vi "ConnectToISU.vi"(0 "ClientRef_In":refnum<k24>, 5 "error in (no error)":errorcluster, 6 "hostName":string="localhost", 8 "portNum":i32=50501, 9 "Get FWver(t)":bool, 11 "RunStartTest(T)":bool) -> (10 "StartTest?(P/F)":bool, 12 "GetVersion":string, 14 "ClientRef_out":refnum<k24>, 16 "ElapsedTime(s)":dbl format="%#.6g", 19 "error out":errorcluster)   [LabVIEW 2018]
uses:
  C:/RageATE-Tetra/Support/TetraLabGUI/FieldTestClient.dll
  Support/TetraLabGUI/FieldTestClient.dll
panel:
  out "FwVer(str)":string
  out "NaN/Path/Refnum?":bool
  out "StartTime":dbl format="%#.6f"
  out "Close?":bool
  out "isu_connected?(t)":bool
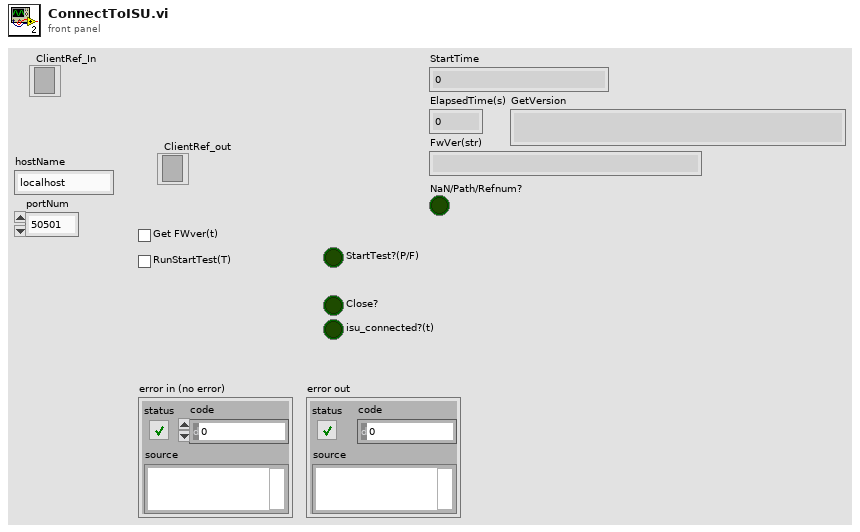
[diagram p1: front panel]
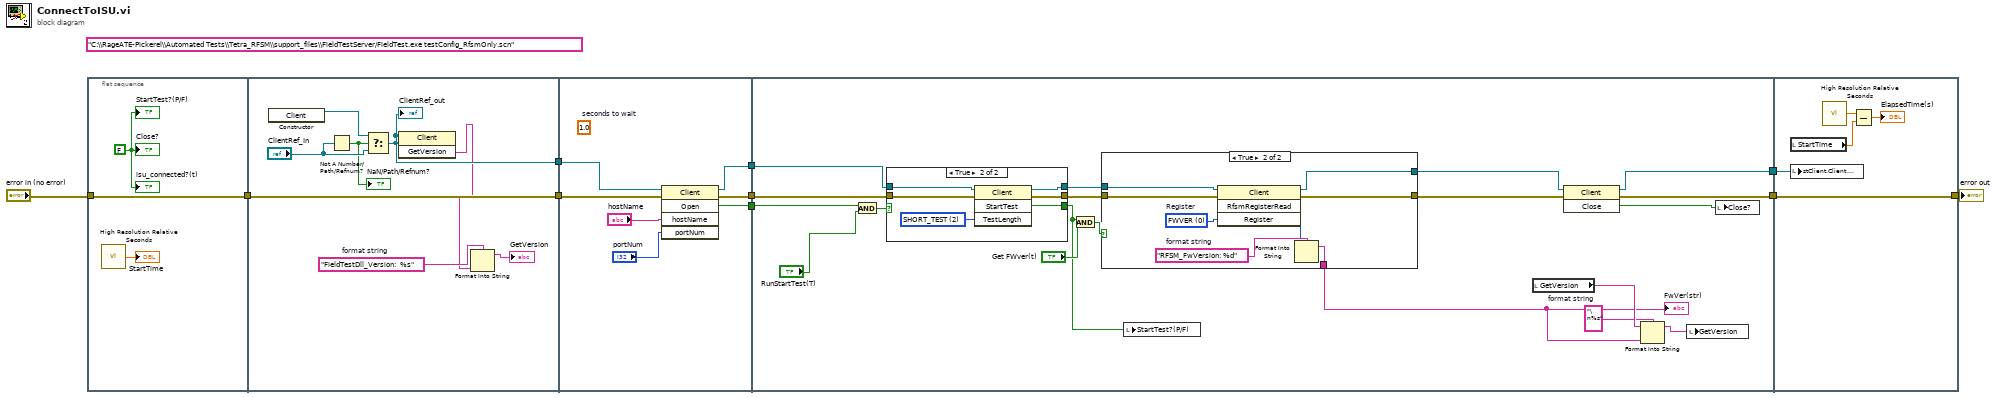
[diagram p0: block diagram]
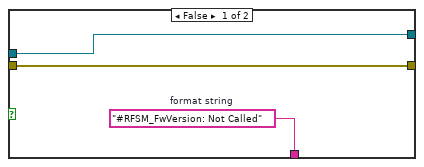
[diagram p2: hidden frame]
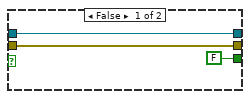
[diagram p3: hidden frame]
diagram:
  (unwired) "C:\\RageATE-Pickerel\\Automated Tests\\Tetra_RFSM\\support_files\\FieldTestServer/FieldTest.exe testConfig_RfsmOnly.scn" ("command line")
  n1 = flat-sequence {
    tunnel: "error in (no error)" -> [w13]
    tunnel: [w13] -> w4
    tunnel: [w21] -> w7
    tunnel: w4 -> [w21]
    tunnel: [w18] -> w1
    tunnel: [w24] -> w10
    tunnel: [w25] -> w9
    tunnel: [w27] -> w8
    tunnel: w7 -> [w28]
    tunnel: w1 -> [w26]
    tunnel: w10 -> [w46]
    tunnel: w9 -> [w47]
    tunnel: w8 -> [w42]
    tunnel: [w29] -> w3
    tunnel: [w45] -> w2
    tunnel: [w72] -> w6
    tunnel: w3 -> [w72]
    tunnel: w2 -> [w68]
    frame #0 {
      w12 = FALSE
      n2 = call <vilib>:"High Resolution Relative Seconds.vi"() -> ("relative seconds"=→"StartTime":dbl)
      "isu_connected?(t)" <- w12
      "Close?" <- w12
      "StartTest?(P/F)" <- w12
    }
    frame #1 {
      w16 = "FieldTestDll_Version:  %s"  # format string
      n3 = constructor class="Client"() -> (reference out=w20:refnum<k24>)  [unwired: 3 in, 2 out]
      n4 = Not A Number/Path/Refnum?(number/path/refnum="ClientRef_In") -> (NaN/Path/Refnum?=w17:bool)
      "NaN/Path/Refnum?" <- w17
      n5 = Select(t=w20, s=w17, f="ClientRef_In") -> (s? t:f=w18:refnum<k24>)
      "ClientRef_out" <- w18
      n6 = invoke class="Client" method="GetVersion"(reference=w18) -> ("GetVersion"=w15:string)  [unwired: 2 in, 2 out]
      n7 = Format Into String(format string=w16, w15) -> (resulting string=→"GetVersion":string)  [unwired: 2 in, 1 out]
    }
    frame #2 {
      (unwired) 1.0  # seconds to wait
      n8 = invoke class="Client" method="Open"(reference=w26, error in=w28, "hostName"="hostName", "portNum"="portNum") -> (reference out=w25:refnum<k24>, error out=w24:errorcluster, "Open"=w27:bool)  [unwired: 1 in, 2 out]
    }
    frame #3 {
      w34 = "\n%s"  # format string
      n9 = And(x=w42, y="RunStartTest(T)") -> (x .and. y?=w43:bool)
      n10 = case shown="True" w43 {
        tunnel: w46 -> [w60 w66]
        tunnel: w47 -> [w61 w65]
        tunnel: [w61 w62] -> w41
        tunnel: [w60 w64] -> w40
        tunnel: [FALSE ("StartTest") w63] -> w30
        frame False {
        }
        frame True {
          w67 = 2 items=["FULL_TEST"=1, "SHORT_TEST"=2] ("TestLength")
          n11 = invoke class="Client" method="StartTest"(reference=w65, error in=w66, "TestLength"=w67) -> (reference out=w62:refnum<k24>, error out=w64:errorcluster, "StartTest"=w63:bool)  [unwired: 1 in, 1 out]
        }
      }
      n12 = And(x=w30, y="Get FWver(t)") -> (x .and. y?=w37:bool)
      n13 = case shown="True" w37 {
        tunnel: w41 -> [w50 w57]
        tunnel: w40 -> [w49 w52]
        tunnel: [w49 w51] -> w39
        tunnel: [w50 w56] -> w38
        tunnel: [w48 w53] -> w33
        frame False {
          w48 = "#RFSM_FwVersion: Not Called"  # format string
        }
        frame True {
          w55 = "RFSM_FwVersion: %d"  # format string
          w58 = 0 items=["FWVER", "STATUS", "FREQ_COUNT", "CTRL", "RETRACE_TIME", "TABLE_DEPTH", "MSCANLINES", "SOS_COUNTER", "FILTER_SWITCH", "VTUNE", "GATETIME", "MUTE1", "MUTE2", "MUTE3", "MUTE4", "MUTE5", "MUTE6", "MUTE7", "MUTE8", "MUTE9", "MUTE10", "MUTE11", "MUTE12", "MUTE13", "MUTE14", "MUTE15", "MUTE16", "MUTE17", "MUTE18", "MUTE19", "MUTE20", "SWITCH0", "SWITCH1", "SWITCH2", "SWITCH3", "SWITCH4", "SWITCH5", "SWITCH6", "SWITCH7", "SWITCH8", "SWITCH9", "SOS_DELAY", "CURRENT_TEMPERATURE"]  # Register
          n14 = invoke class="Client" method="RfsmRegisterRead"(reference=w57, error in=w52, "Register"=w58) -> (reference out=w56:refnum<k24>, error out=w51:errorcluster, "RfsmRegisterRead"=w54:i32)  [unwired: 1 in, 1 out]
          n15 = Format Into String(format string=w55, w54) -> (resulting string=w53:string)  [unwired: 2 in, 1 out]
        }
      }
      "FwVer(str)" <- w33
      n16 = local write "StartTest?(P/F)"(w30) -> ()
      n17 = local read "GetVersion"() -> (w35:string)
      n18 = invoke class="Client" method="Close"(reference=w38, error in=w39) -> (reference out=w45:refnum<k24>, error out=w29:errorcluster, "Close"=w44:bool)  [unwired: 1 in]
      n19 = Format Into String(format string=w34, initial string=w35, w33) -> (resulting string=w32:string)  [unwired: 1 in, 1 out]
      n20 = local write "GetVersion"(w32) -> ()
      n21 = local write "Close?"(w44) -> ()
    }
    frame #4 {
      n22 = local read "StartTime"() -> (w70:dbl)
      n23 = local write "ClientRef_out"(w68) -> ()
      n24 = call <vilib>:"High Resolution Relative Seconds.vi"() -> ("relative seconds"=w71:dbl)
      n25 = Subtract(x=w71, y=w70) -> (x-y=→"ElapsedTime(s)":dbl)
    }
  }
  "error out" <- w6
